vi "GetParentLayerName.vi"(8 "error in (no error)":errorcluster, 11 "CDependencyItemRule in":refnum<class "CDependencyItemRule.lvclass">) -> (0 "error out":errorcluster, 1 "Parent layer name":string, 3 "CDependencyItemRule out":refnum<class "CDependencyItemRule.lvclass">)   [LabVIEW 2020, in "LabVIEWContainers.lvlib" / "CDependencyItemRule.lvclass"]
uses:
  CDependencyItemRule.lvclass
  CDependencyItemRule.lvclass/CDependencyItemRule.ctl
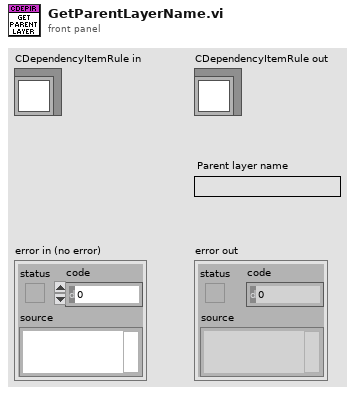
[diagram p1: front panel]
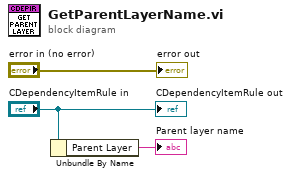
[diagram p0: block diagram]
diagram:
  n1 = Unbundle By Name("CDependencyItemRule in") -> ("Parent Layer"=→"Parent layer name":string)
  "error out" <- "error in (no error)"
  "CDependencyItemRule out" <- "CDependencyItemRule in"
